vi "通信状态入队列.vi"(8 "错误输入（无错误）":errorcluster, 10 "发送报文":string, 11 "枚举":enum16{"打开连接", "发送数据", "读取数据", "数据处理", "关闭连接"}(ring)) -> (0 "错误输出":errorcluster)   [LabVIEW 2016, in "数据传输系统-03.lvlib"]
panel:
  out "data":T1
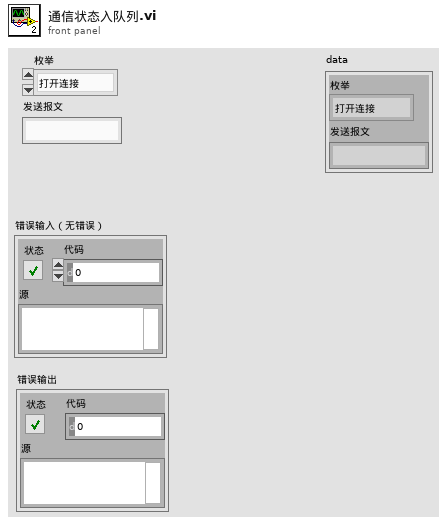
[diagram p1: front panel]
types:
  T1 = cluster{"枚举":enum16{"打开连接", "发送数据", "读取数据", "数据处理", "关闭连接"}, "发送报文":string}
  T2 = cluster{"setini":string, "sysini":string, "hechaini":string, "actualwrite":string, "actualread":string, "datasent":string, "反控命令信息队列":string, "反控与仪器交互":string}
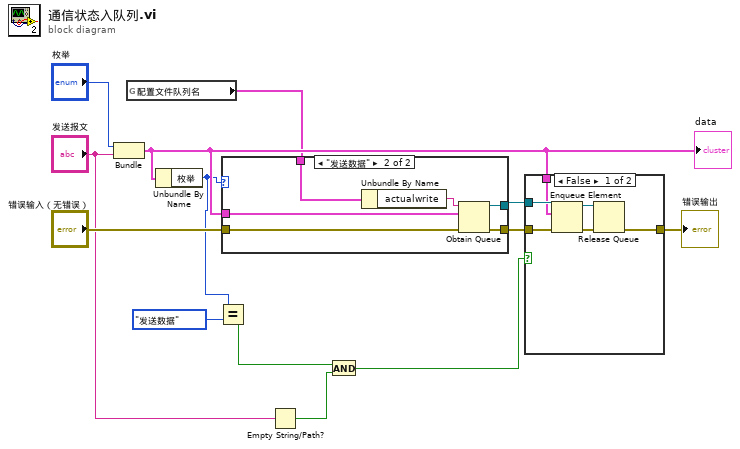
[diagram p0: block diagram]
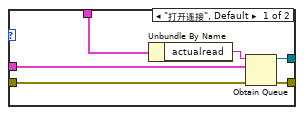
[diagram p3: hidden frame]
diagram:
  n1 = Bundle("枚举"="枚举", "发送报文"="发送报文") -> (w8:T1)  [unwired: 1 in]
  "data" <- w8
  n2 = global read "全局1.vi" "配置文件队列名"() -> (w7:T2)
  n3 = Unbundle By Name(w8) -> ("枚举"=w5:enum16{"打开连接", "发送数据", "读取数据", "数据处理", "关闭连接"})
  n4 = Equal?(x=w5, y=enum16{"打开连接", "发送数据", "读取数据", "数据处理", "关闭连接"}."发送数据") -> (x = y?=w2:bool)
  n5 = case shown="\"发送数据\"" w5 {
    tunnel: [w19 w25] -> w13
    tunnel: [w18 w24] -> w12
    tunnel: "错误输入（无错误）" -> [w17 w23]
    tunnel: w8 -> [w15 w21]
    tunnel: w7 -> [w14 w20]
    frame "打开连接", Default {
      n6 = Unbundle By Name(w14) -> ("actualread"=w16:string)
      n7 = Obtain Queue(name (unnamed)=w16, element data type=w15, error in (no error)=w17) -> (queue out=w19:refnum<queue>, error out=w18:errorcluster)  [unwired: 2 in, 1 out]
    }
    frame "发送数据" {
      n8 = Unbundle By Name(w20) -> ("actualwrite"=w22:string)
      n9 = Obtain Queue(name (unnamed)=w22, element data type=w21, error in (no error)=w23) -> (queue out=w25:refnum<queue>, error out=w24:errorcluster)  [unwired: 2 in, 1 out]
    }
  }
  n10 = Empty String/Path?(string/path="发送报文") -> (empty?=w3:bool)
  n11 = And(x=w2, y=w3) -> (x .and. y?=w1:bool)
  n12 = case shown="False" w1 {
    tunnel: w13 -> [w30 _]
    tunnel: w12 -> [w29 w32]
    tunnel: [w27 w32] -> w10
    tunnel: w8 -> [w26 _]
    frame False {
      n13 = Enqueue Element(queue=w30, element=w26, error in (no error)=w29) -> (queue out=w31:refnum<queue>, error out=w28:errorcluster)  [unwired: 1 in, 1 out]
      n14 = Release Queue(queue=w31, error in (no error)=w28) -> (error out=w27:errorcluster)  [unwired: 1 in, 2 out]
    }
    frame True {
    }
  }
  "错误输出" <- w10
